vi "EmergencyFormatString (1).vi"(11 "Array":bool[](array[boolean])) -> ()   [LabVIEW 2017]
uses:
  EmergencyStringGLOBAL.vi
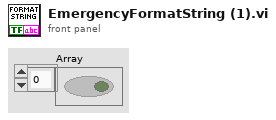
[diagram p1: front panel]
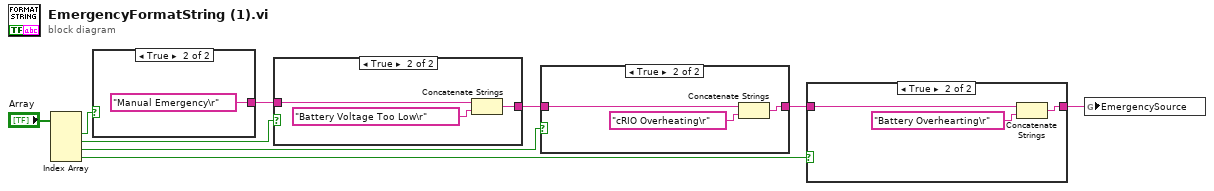
[diagram p0: block diagram]
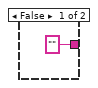
[diagram p5: hidden frame]
diagram:
  n1 = Index Array(array="Array") -> (element #1=w8:bool, element #2=w3:bool, element #3=w2:bool, element #4=w1:bool)  [unwired: 4 in]
  n2 = case shown="True" w8 {
    tunnel: ["" ("EmergencySource") "Manual Emergency\r" ("EmergencySource")] -> w7
    frame False {
    }
    frame True {
    }
  }
  n3 = case shown="True" w3 {
    tunnel: w7 -> [w12 w14]
    tunnel: [w12 w13] -> w6
    frame False {
    }
    frame True {
      n4 = Concatenate Strings(w14, "Battery Voltage Too Low\r" ("EmergencySource")) -> (w13:string)
    }
  }
  n5 = case shown="True" w2 {
    tunnel: w6 -> [w16 w18]
    tunnel: [w16 w17] -> w5
    frame False {
    }
    frame True {
      n6 = Concatenate Strings(w18, "cRIO Overheating\r" ("EmergencySource")) -> (w17:string)
    }
  }
  n7 = case shown="True" w1 {
    tunnel: w5 -> [w20 w22]
    tunnel: [w20 w21] -> w4
    frame False {
    }
    frame True {
      n8 = Concatenate Strings(w22, "Battery Overhearting\r" ("EmergencySource")) -> (w21:string)
    }
  }
  n9 = global write "EmergencyStringGLOBAL.vi" "EmergencySource"(w4) -> ()
